vi "QPD config globals.vi"() -> ()   [LabVIEW 2016]
panel:
  in  "maximum value":dbl=10.0 format="%0.2f"
  in  "minimum value":dbl=-10.0
  in  "Sampling rate (s-1)":dbl=100.0 format="%0.2f"
  in  "A-to-D channels\nfor x, y, power, supply":tag="Dev1/ai2, Dev1/ai4, Dev1/ai0"
  # "Configure QPD hardware here.  Remember to save as default."
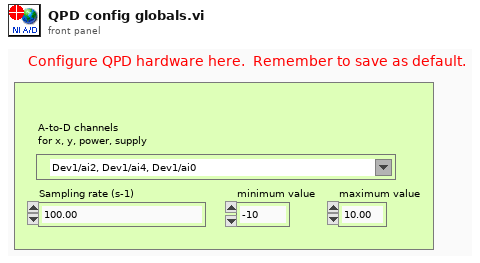
[diagram p1: front panel]
diagram:
